vi "AcqPtEtalonnage.vi"(4 "entrée d'erreur":errorcluster caption="entrée d'erreur (pas d'erreur)", 7 "Projet":string) -> (0 "sortie d'erreur":errorcluster)   [LabVIEW 2017]
uses:
  <vilib>/Analysis/NI_AALBase.lvlib
  DefDeType/WhichPath.ctl
panel:
  out "fichier :":path
  out "Glissière":i32(slide) scale=0.0..300.0
  out "tableau ajouté":dbl[](array[numeric]) format="%#.5f"
  out "Ecart-type":dbl[](array[numeric])
  out "Moy":dbl[](array[numeric]) format="%#.5f"
  out "ApercuMesures":dbl[](array[numeric])
  # "Acquisition d'un point d'étalonnage"
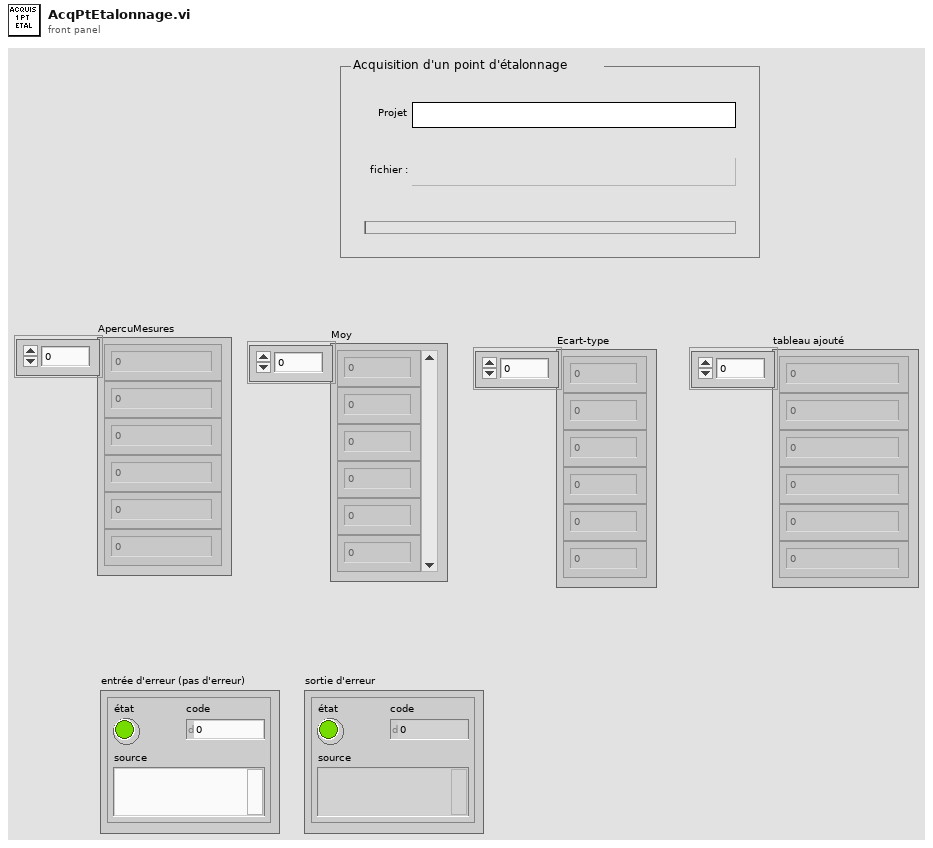
[diagram p1: front panel]
types:
  T1 = typedef "WhichPath.ctl" = enum16{"DossierProjet", "Config", "Meas", "MeasPCI", "MeasCRIO1", "MeasCRIO2", "MeasQualisys", "MeasHBM", "MeasTDMS", "Fig", "Res"}
  T2 = enum16{"open", "replace", "create", "open or create", "replace or create", "replace or create with confirmation"}
  T3 = typedef "ConfigTotale.ctl" = cluster{"VoltageChannels":T4, "WheastoneBridgeChannels":T5, "Configuration":T6}
  T4 = typedef "VoltageChannels.ctl" = cluster{"ChannelNames":string[], "Sensitivity(Unit/V)":dbl[], "AutoZero":bool[], "ChannelUnits":string[], "Offsets(Units)":dbl[], "Graph Num":u8[]}
  T5 = typedef "WBridgeChannels.ctl" = cluster{"ChannelNames":string[], "Sensitivity(Unit/V)":dbl[], "AutoZero":bool[], "ChannelUnits":string[], "Offsets(Units)":dbl[], "Graph Num":u8[]}
  T6 = typedef "Configuration.ctl" = cluster{"AcqSamplingRate(Hz)":u32, "AcqTime(s)":u32, "Trigger":bool, "NbVoltageChannels":u32, "NbWBridgeChannels":u32, "Qualisys":bool, "Hexapode":bool, "FinalSamplingRate(Hz)":u32, "QualisysDataType":enum16{"6DOF", "3DTracking", "6DOF + 3D"}, "Nortek":bool, "HBM":bool}
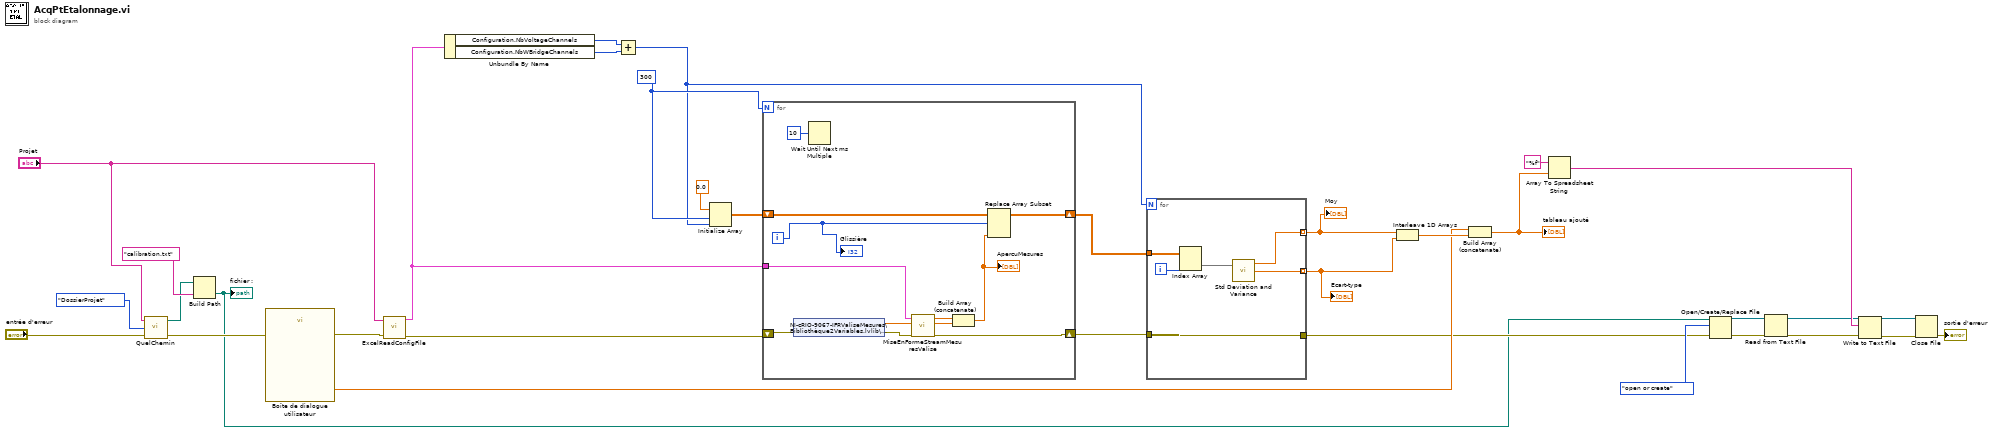
[diagram p0: block diagram]
diagram:
  w30 = 300 ("taille de la dimension")
  n1 = call "QuelChemin.vi"("Entrée d'erreur"="entrée d'erreur", "WhichPath?"=WhichPath."DossierProjet", "NomProjet"="Projet") -> ("Sortie d'erreur"=w5:errorcluster, "SurDisqueLocal"=w2:path)  [unwired: 1 out]
  n2 = Build Path(base path=w2, name or relative path="calibration.txt" ("nom ou chemin relatif")) -> (appended path=w1:path)
  "fichier :" <- w1
  n3 = call "Boîte de dialogue utilisateur"("error in (no error)"=w5) -> ("ValRef"=w20:dbl, "error out"=w29:errorcluster)  [unwired: 16 in, 1 out]
  n4 = call "ExcelReadConfigFile.vi"("NomProjet"="Projet", "error in (no error)"=w29) -> ("ConfigurationTotale"=w27:T3, "error out"=w28:errorcluster)  [unwired: 3 in]
  n5 = Unbundle By Name(w27) -> ("Configuration.NbVoltageChannels"=w26:u32, "Configuration.NbWBridgeChannels"=w25:u32)
  n6 = Add(x=w26, y=w25) -> (x+y=w24:u32)
  n7 = Initialize Array(0.0 ("élément"), w30, w24) -> (w33:dbl[][])
  n8 = for {
    N: w30 -> [_]
    shift-right: [w41] -> w32
    shift-left: w28 -> [w45]
    shift-right: [w43] -> w31
    shift-left: w33 -> [w44]
    tunnel: w27 -> [w39]
    i -> [w35]
    n9 = shared-variable "NI-cRIO-9067-IFRValiseMesures\\Bibliothèque2Variables.lvlib\\ApercuMesures"(error in=w45) -> (w40:dbl[], error out=w42:errorcluster)
    n10 = Wait Until Next ms Multiple(millisecond multiple=u32 10 ("n millisecondes")) -> ()  [unwired: 1 out]
    n11 = call "MiseEnFormeStreamMesuresValise.vi"("Error In"=w42, "MesuresBrutesValise"=w40, "ConfigTotale"=w39) -> ("Error Out"=w41:errorcluster, "VoltageChannels1(0to15)"=w37:dbl[], "WBridgeChannels"=w38:dbl[])  [unwired: 2 in]
    n12 = Build Array (concatenate)(w38, w37) -> (w36:dbl[])
    "ApercuMesures" <- w36
    n13 = Replace Array Subset(array=w44, new element=w36, index (row)=w35) -> (w43:dbl[][])  [unwired: 1 in]
    "Glissière" <- w35
  }
  n14 = for {
    N: w24 -> [_]
    tunnel: w32 -> [w52]
    tunnel: [w52] -> w8
    tunnel: [w51] -> w23 mode=indexing
    tunnel: [w50] -> w22 mode=indexing
    tunnel: w31 -> [w49]
    i -> [w48]
    n15 = Index Array(array=w49, index (col)=w48) -> (element=w47:dbl[])  [unwired: 1 in]
    n16 = call <vilib>:"Std Deviation and Variance.vi"("X"=w47) -> ("mean"=w51:dbl, "standard deviation"=w50:dbl)  [unwired: 1 in, 1 out]
  }
  "Moy" <- w23
  "Ecart-type" <- w22
  n17 = Interleave 1D Arrays(w23, w22) -> (w21:dbl[])
  n18 = Build Array (concatenate)(w20, w21) -> (w18:dbl[])
  "tableau ajouté" <- w18
  n19 = Array To Spreadsheet String(array=w18, 3:"%f" ("chaîne de format")) -> (spreadsheet string=w14:string)  [unwired: 1 in]
  n20 = Open/Create/Replace File(file path (use dialog)=w1, error in=w8, operation (0:open)=T2."open or create" ("opération (0 : open)")) -> (refnum out=w11:refnum<file>, error out=w10:errorcluster)  [unwired: 3 in, 1 out]
  n21 = Read from Text File(file (use dialog)=w11, error in=w10) -> (refnum out=w12:refnum<file>, error out=w13:errorcluster)  [unwired: 2 in, 2 out]
  n22 = Write to Text File(file (use dialog)=w12, text=w14, error in=w13) -> (refnum out=w15:refnum<file>, error out=w16:errorcluster)  [unwired: 1 in, 1 out]
  n23 = Close File(refnum=w15, error in=w16) -> (error out=→"sortie d'erreur":errorcluster)  [unwired: 1 out]
